vi "Set Torque Setpoint.vi"(8 "error in (no error)":errorcluster, 10 "CCW torque (Nm)":dbl, 11 "NI_Robotics_KUKA youBot Arm Motor in":refnum<class "NI_Robotics_KUKA youBot Arm Motor.lvclass">) -> (0 "error out":errorcluster, 3 "NI_Robotics_KUKA youBot Arm Motor out":refnum<class "NI_Robotics_KUKA youBot Arm Motor.lvclass">)   [LabVIEW 2017, in "NI_Robotics_KUKA youBot Host.lvlib" / "NI_Robotics_KUKA youBot Arm Motor.lvclass"]
uses:
  <vilib>/robotics/KUKA youBot/Motor/Arm Motor/NI_Robotics_KUKA youBot Arm Motor.lvclass
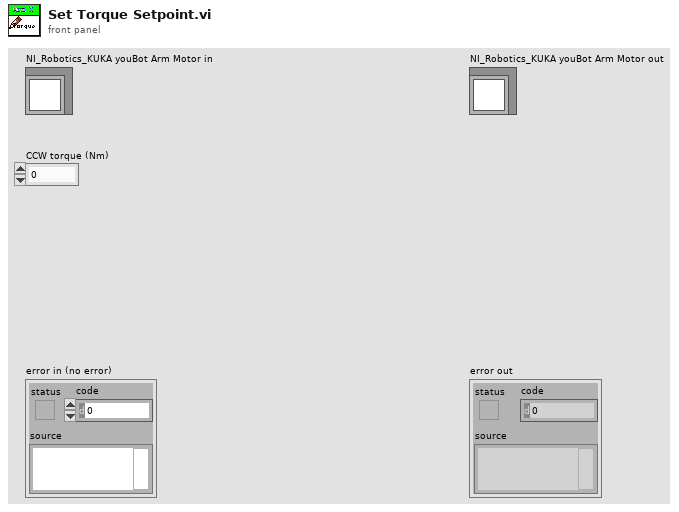
[diagram p1: front panel]
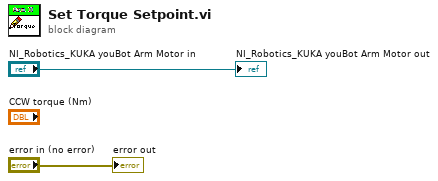
[diagram p0: block diagram]
diagram:
  "error out" <- "error in (no error)"
  "NI_Robotics_KUKA youBot Arm Motor out" <- "NI_Robotics_KUKA youBot Arm Motor in"
